vi "fit 3 section stuckbead-v2.vi"(2 "Calib-QPD scan (V)":dbl[](array[numeric]), 3 "X=T; Y=F":bool, 4 "Calib-stage position (um)":dbl[](array[numeric])) -> (0 "(1+2+3) stuckbead-scan coefficient":T1 {"(3)stuckbead-scan coefficient" min=0.0 max=127.0 format="%#.2f"; "(2)stuckbead-scan coefficient" min=0.0 max=127.0 format="%#.2f"; "(1)stuckbead-scan coefficient" min=0.0 max=127.0 format="%#.2f"}, 1 "best fit position out":dbl[](array[numeric]))   [LabVIEW 2014]
uses:
  (1+2+3)fit stuckbead coefficient.ctl
  <vilib>/Analysis/polynomials.llb/Scalar Polynomial Evaluation (DBL).vi
  <vilib>/Analysis/NI_AALPro.lvlib
panel:
  out "bead position out (nm)":dbl[](array[numeric])
  out "center of position (um)":dbl
  out "P(a)":dbl
  in  "a":dbl
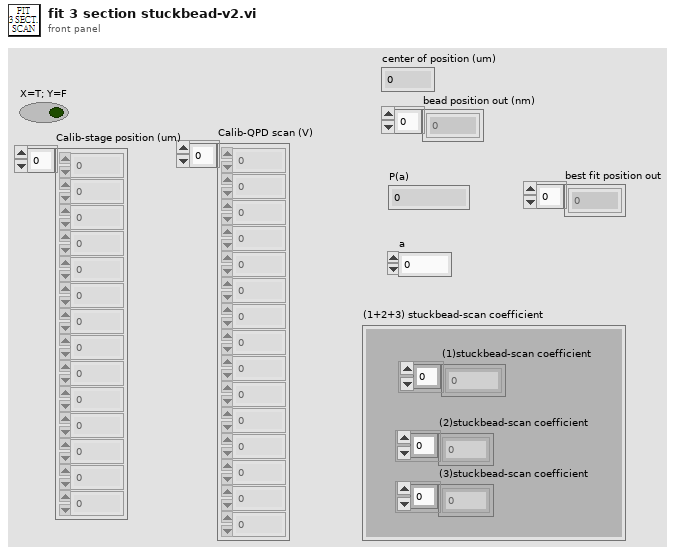
[diagram p1: front panel]
types:
  T1 = typedef "(1+2+3)fit stuckbead coefficient.ctl" = cluster{"(1)stuckbead-scan coefficient ":dbl[], "(2)stuckbead-scan coefficient ":dbl[], "(3)stuckbead-scan coefficient":dbl[]}
  T2 = cluster{"Polynomial Coefficients":dbl[], "Polynomial Coefficients":dbl[], "Polynomial Coefficients":dbl[]}
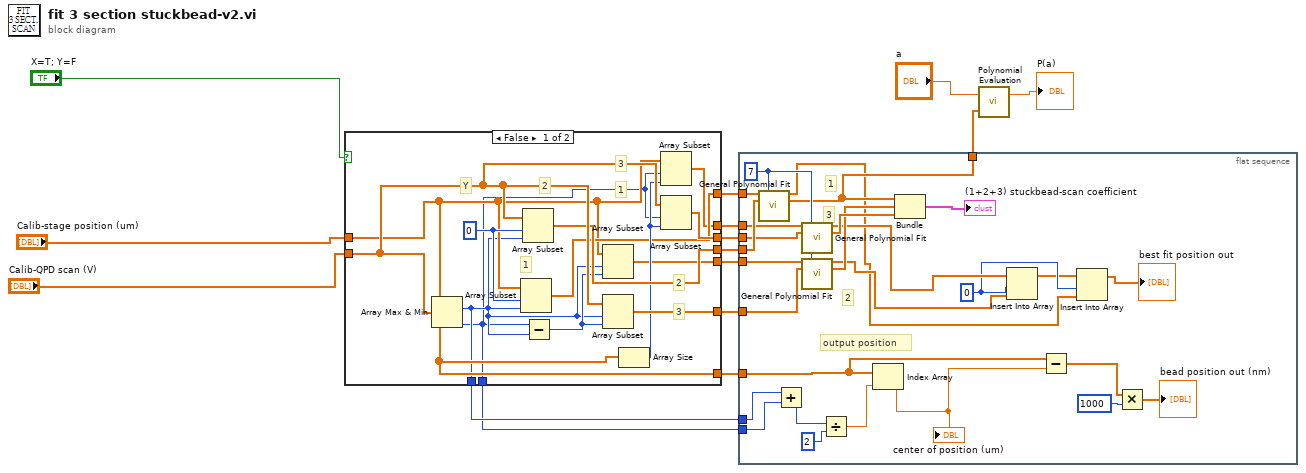
[diagram p0: block diagram]
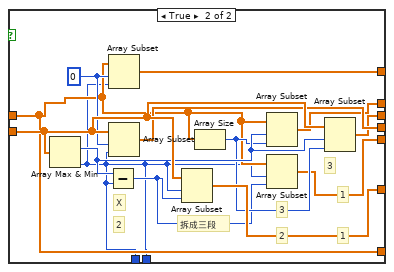
[diagram p2: hidden frame]
diagram:
  n1 = case shown="False" "X=T; Y=F" {
    tunnel: "Calib-QPD scan (V)" -> [w28 w41]
    tunnel: [w27 w40] -> w14
    tunnel: [w26 w39] -> w15
    tunnel: [w25 w38] -> w13
    tunnel: "Calib-stage position (um)" -> [w18 w30]
    tunnel: [w21 w33] -> w12
    tunnel: [w20 w32] -> w11
    tunnel: [w19 w31] -> w10
    tunnel: [w18 w30] -> w3
    tunnel: [w17 w29] -> w2
    tunnel: [w16 w29] -> w1
    frame False {
      w24 = 0 ("index")
      # "2"
      # "3"
      # "1"
      # "Y"
      # "3"
      # "2"
      # "1"
      n2 = Array Max & Min(array=w28) -> (max index (indices)=w17:i32, min index (indices)=w16:i32)  [unwired: 2 out]
      n3 = Array Subset(array=w18, index=w24, length=w17) -> (w21:dbl[])
      n4 = Array Subset(array=w28, index=w24, length=w17) -> (w27:dbl[])
      n5 = Subtract(x=w16, y=w17) -> (x-y=w22:i32)
      n6 = Array Subset(array=w18, index=w17, length=w22) -> (w20:dbl[])
      n7 = Array Subset(array=w28, index=w17, length=w22) -> (w26:dbl[])
      n8 = Array Size(array=w18) -> (size(s)=w23:i32)
      n9 = Array Subset(array=w18, index=w16, length=w23) -> (w19:dbl[])
      n10 = Array Subset(array=w28, index=w16, length=w23) -> (w25:dbl[])
    }
    frame True {
      w37 = 0 ("index")
      # "3"
      # "2"
      # "1"
      # "拆成三段"
      # "X"
      # "3"
      # "2"
      # "1"
      n11 = Array Max & Min(array=w41) -> (max index (indices)=w36:i32, min index (indices)=w29:i32)  [unwired: 2 out]
      n12 = Subtract(x=w36, y=w29) -> (x-y=w34:i32)
      n13 = Array Subset(array=w30, index=w37, length=w29) -> (w33:dbl[])
      n14 = Array Subset(array=w41, index=w37, length=w29) -> (w40:dbl[])
      n15 = Array Subset(array=w41, index=w29, length=w34) -> (w39:dbl[])
      n16 = Array Size(array=w30) -> (size(s)=w35:i32)
      n17 = Array Subset(array=w30, index=w36, length=w35) -> (w31:dbl[])
      n18 = Array Subset(array=w30, index=w29, length=w34) -> (w32:dbl[])
      n19 = Array Subset(array=w41, index=w36, length=w35) -> (w38:dbl[])
    }
  }
  n20 = flat-sequence {
    tunnel: w15 -> [w68]
    tunnel: w14 -> [w67]
    tunnel: w13 -> [w66]
    tunnel: w12 -> [w65]
    tunnel: w11 -> [w64]
    tunnel: w10 -> [w63]
    tunnel: [w58] -> w6
    tunnel: w3 -> [w46]
    tunnel: w2 -> [w50]
    tunnel: w1 -> [w49]
    frame #0 {
      w55 = 0 ("index")
      w59 = 7 ("polynomial order")
      # "output position"
      # "3"
      # "2"
      # "1"
      n21 = call <vilib>:"General Polynomial Fit.vi"("Y"=w65, "polynomial order"=w59, "X"=w67) -> ("Best Polynomial Fit"=w53:dbl[], "Polynomial Coefficients"=w58:dbl[])  [unwired: 9 in, 2 out]
      n22 = Add(x=w50, y=w49) -> (x+y=w51:i32)
      n23 = call <vilib>:"General Polynomial Fit.vi"("Y"=w63, "polynomial order"=w59, "X"=w66) -> ("Best Polynomial Fit"=w57:dbl[], "Polynomial Coefficients"=w62:dbl[])  [unwired: 9 in, 2 out]
      n24 = call <vilib>:"General Polynomial Fit.vi"("Y"=w64, "polynomial order"=w59, "X"=w68) -> ("Best Polynomial Fit"=w56:dbl[], "Polynomial Coefficients"=w60:dbl[])  [unwired: 9 in, 2 out]
      n25 = Divide(x=w51, y=2) -> (x/y=w47:dbl)
      n26 = Index Array(array=w46, index=w47) -> (element=w45:dbl)
      "center of position (um)" <- w45
      n27 = Bundle("Polynomial Coefficients"=w58, "Polynomial Coefficients"=w60, "Polynomial Coefficients"=w62) -> (→"(1+2+3) stuckbead-scan coefficient":T2)  [unwired: 1 in]
      n28 = Insert Into Array(array=w57, index=w55, new element=w56) -> (w54:dbl[])
      n29 = Subtract(x=w46, y=w45) -> (x-y=w44:dbl[])
      n30 = Insert Into Array(array=w54, index=w55, new element=w53) -> (→"best fit position out":dbl[])
      n31 = Multiply(x=w44, y=1000) -> (x*y=→"bead position out (nm)":dbl[])
    }
  }
  n32 = call-poly <vilib>:"Polynomial Evaluation.vi"("P(x)"=w6, "a"="a") -> ("P(a)"=→"P(a)":dbl)  [unwired: 1 out]
